vi "Set Cursor.vi"(9 "icon":u16, 11 "MainController.lvclass":refnum<class "MainController.lvclass">) -> ()   [LabVIEW 2012, in "Win8uiFramework.lvlib" / "MainController.lvclass"]
uses:
  MainController.lvclass
  ViewableActor.lvclass/ViewableActor.ctl
  Read UI VI Ref.vi
  <vilib>/Utility/cursorutil.llb/Set Cursor (Icon Pict).vi
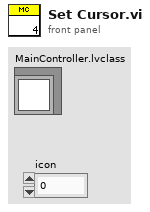
[diagram p1: front panel]
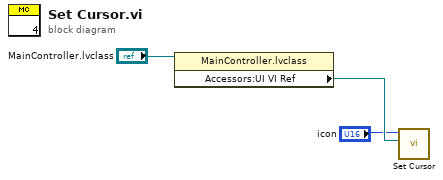
[diagram p0: block diagram]
diagram:
  n1 = property class="MainController.lvclass"(reference="MainController.lvclass") -> ("Accessors:UI VI Ref"=w2:refnum<vi>)  [unwired: 1 in, 2 out]
  n2 = call-poly <vilib>:"Set Cursor.vi"("VI reference (current VI)"=w2, "icon"="icon") -> ()  [unwired: 8 in, 2 out]
